vi "hotSpotsD2T.vi"(2 "Hotspot Number":i32, 3 "Basket Number":i32) -> (0 "rotation angle":dbl, 1 "distance to basket":dbl)   [LabVIEW 2011]
panel:
  # "z"
  # "R"
  # "Our Basket"
  # "yField"
  # "1"
  # "3"
  # "2"
  # "4"
  # "xField"
  # "xRobot"
  # "r"
  # "yRobot"
  # "y"
  # "x"
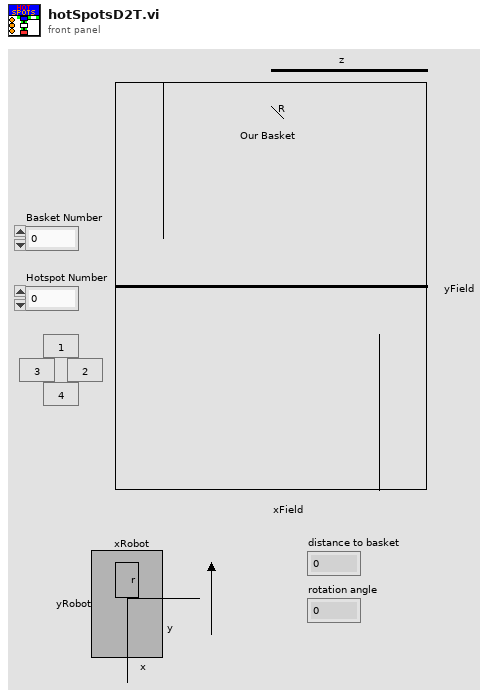
[diagram p1: front panel]
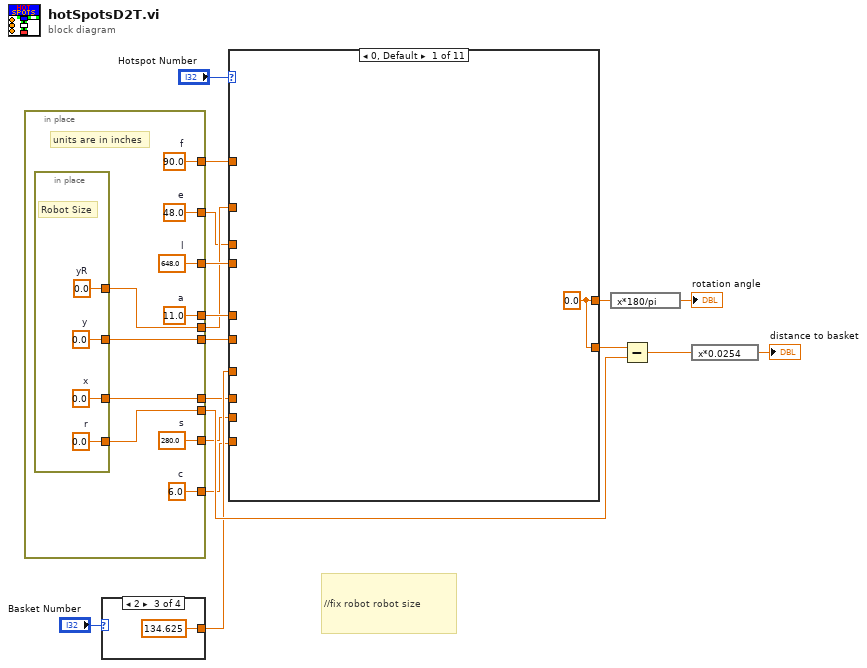
[diagram p0: block diagram]
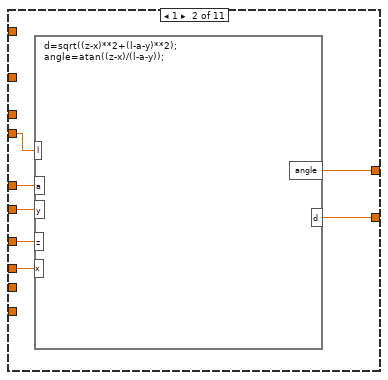
[diagram p2: hidden frame]
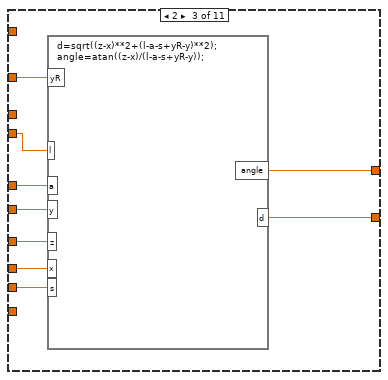
[diagram p3: hidden frame]
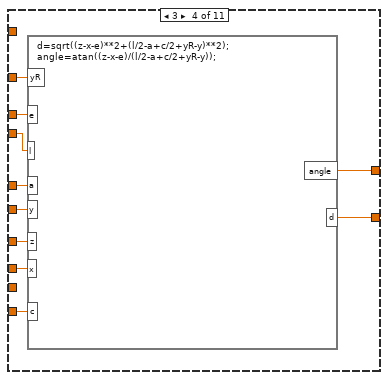
[diagram p4: hidden frame]
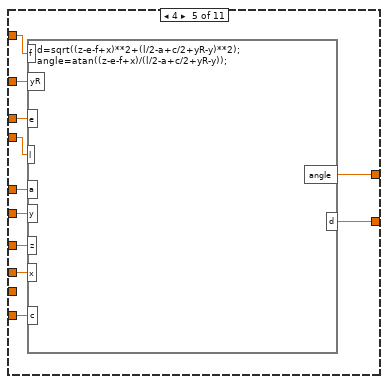
[diagram p5: hidden frame]
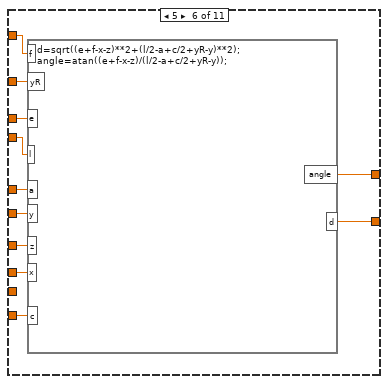
[diagram p6: hidden frame]
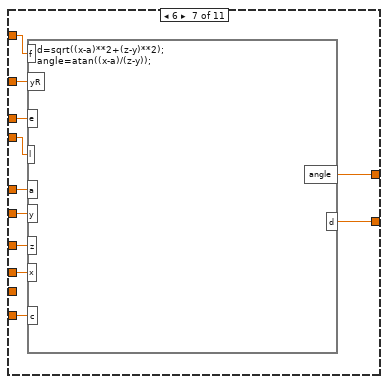
[diagram p7: hidden frame]
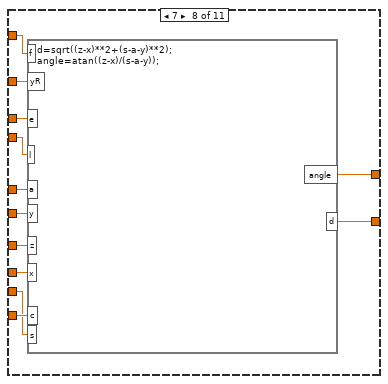
[diagram p8: hidden frame]
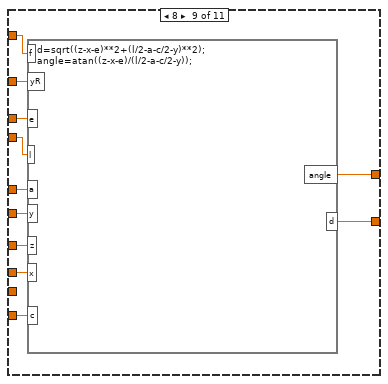
[diagram p9: hidden frame]
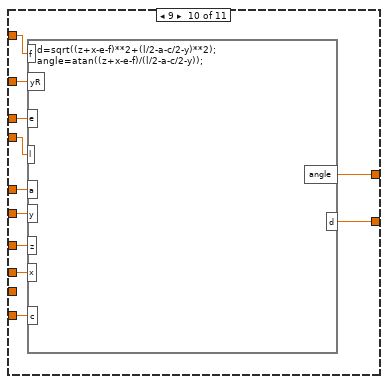
[diagram p10: hidden frame]
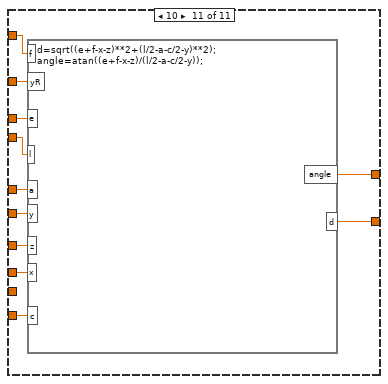
[diagram p11: hidden frame]
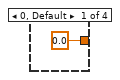
[diagram p12: hidden frame]
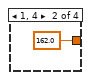
[diagram p13: hidden frame]
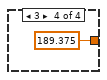
[diagram p14: hidden frame]
diagram:
  # "//fix robot robot size"
  n1 = in-place {
    in-place-border: [w28] -> w11
    in-place-border: [w27] -> w10
    in-place-border: [w26] -> w9
    in-place-border: [w25] -> w8
    in-place-border: [w24] -> w6
    in-place-border: [w23] -> w5
    in-place-border: [w22] -> w4
    in-place-border: [w21] -> w3
    in-place-border: [w20] -> w2
    in-place-border: [w19] -> w1
    w19 = 90.0  # f
    w21 = 6.0  # c
    w20 = 48.0  # e
    w23 = 280.0  # s
    w26 = 11.0  # a
    w27 = 648.0  # l
    # "units are in inches"
    n2 = in-place {
      in-place-border: [w32] -> w24
      in-place-border: [w31] -> w22
      in-place-border: [w30] -> w25
      in-place-border: [w29] -> w28
      w32 = 0.0  # x
      w30 = 0.0  # y
      w31 = 0.0  # yR
      w29 = 0.0  # r
      # "Robot Size"
    }
  }
  n3 = case shown="2" "Basket Number" {
    tunnel: [0.0 ("z") 162.0 ("z") 134.625 ("z") 189.375 ("z")] -> w7
    frame 0, Default {
    }
    frame 1, 4 {
    }
    frame 2 {
    }
    frame 3 {
    }
  }
  n4 = case shown="0, Default" "Hotspot Number" {
    tunnel: [w37 w44 w53 w63 w74 w85 w96 w108 w119 w130 w141] -> w13
    tunnel: [w37 w43 w52 w62 w73 w84 w95 w107 w118 w129 w140] -> w12
    tunnel: w10 -> [_ w42 w51 w61 w72 w83 w94 w106 w117 w128 w139]
    tunnel: w9 -> [_ w41 w50 w60 w71 w82 w93 w105 w116 w127 w138]
    tunnel: w8 -> [_ w40 w49 w59 w70 w81 w92 w104 w115 w126 w137]
    tunnel: w7 -> [_ w39 w48 w58 w69 w80 w91 w103 w114 w125 w136]
    tunnel: w6 -> [_ w38 w47 w57 w68 w79 w90 w102 w113 w124 w135]
    tunnel: w5 -> [_ _ w46 _ _ _ _ w97 _ _ _]
    tunnel: w4 -> [_ _ w45 w56 w67 w78 w89 w101 w112 w123 w134]
    tunnel: w3 -> [_ _ _ w55 w66 w77 w88 w100 w111 w122 w133]
    tunnel: w2 -> [_ _ _ w54 w65 w76 w87 w99 w110 w121 w132]
    tunnel: w1 -> [_ _ _ _ w64 w75 w86 w98 w109 w120 w131]
    frame 0, Default {
      w37 = 0.0 ("angle")
    }
    frame 1 {
      n5 = formula code="d=sqrt((z-x)**2+(l-a-y)**2);\nangle=atan((z-x)/(l-a-y));"("l"=w42, "z"=w39, "a"=w41, "x"=w38, "y"=w40) -> ("d"=w44:dbl, "angle"=w43:dbl)
    }
    frame 2 {
      n6 = formula code="d=sqrt((z-x)**2+(l-a-s+yR-y)**2);\nangle=atan((z-x)/(l-a-s+yR-y));"("l"=w51, "z"=w48, "a"=w50, "x"=w47, "y"=w49, "s"=w46, "yR"=w45) -> ("d"=w53:dbl, "angle"=w52:dbl)
    }
    frame 3 {
      n7 = formula code="d=sqrt((z-x-e)**2+(l/2-a+c/2+yR-y)**2);\nangle=atan((z-x-e)/(l/2-a+c/2+yR-y));"("l"=w61, "z"=w58, "a"=w60, "x"=w57, "y"=w59, "c"=w55, "yR"=w56, "e"=w54) -> ("d"=w63:dbl, "angle"=w62:dbl)
    }
    frame 4 {
      n8 = formula code="d=sqrt((z-e-f+x)**2+(l/2-a+c/2+yR-y)**2);\nangle=atan((z-e-f+x)/(l/2-a+c/2+yR-y));"("l"=w72, "z"=w69, "a"=w71, "x"=w68, "y"=w70, "c"=w66, "yR"=w67, "e"=w65, "f"=w64) -> ("d"=w74:dbl, "angle"=w73:dbl)
    }
    frame 5 {
      n9 = formula code="d=sqrt((e+f-x-z)**2+(l/2-a+c/2+yR-y)**2);\nangle=atan((e+f-x-z)/(l/2-a+c/2+yR-y));"("l"=w83, "z"=w80, "a"=w82, "x"=w79, "y"=w81, "c"=w77, "yR"=w78, "e"=w76, "f"=w75) -> ("d"=w85:dbl, "angle"=w84:dbl)
    }
    frame 6 {
      n10 = formula code="d=sqrt((x-a)**2+(z-y)**2);\nangle=atan((x-a)/(z-y));"("l"=w94, "z"=w91, "a"=w93, "x"=w90, "y"=w92, "c"=w88, "yR"=w89, "e"=w87, "f"=w86) -> ("d"=w96:dbl, "angle"=w95:dbl)
    }
    frame 7 {
      n11 = formula code="d=sqrt((z-x)**2+(s-a-y)**2);\nangle=atan((z-x)/(s-a-y));"("l"=w106, "z"=w103, "a"=w105, "x"=w102, "y"=w104, "c"=w100, "yR"=w101, "e"=w99, "f"=w98, "s"=w97) -> ("d"=w108:dbl, "angle"=w107:dbl)
    }
    frame 8 {
      n12 = formula code="d=sqrt((z-x-e)**2+(l/2-a-c/2-y)**2);\nangle=atan((z-x-e)/(l/2-a-c/2-y));"("l"=w117, "z"=w114, "a"=w116, "x"=w113, "y"=w115, "c"=w111, "yR"=w112, "e"=w110, "f"=w109) -> ("d"=w119:dbl, "angle"=w118:dbl)
    }
    frame 9 {
      n13 = formula code="d=sqrt((z+x-e-f)**2+(l/2-a-c/2-y)**2);\nangle=atan((z+x-e-f)/(l/2-a-c/2-y));"("l"=w128, "z"=w125, "a"=w127, "x"=w124, "y"=w126, "c"=w122, "yR"=w123, "e"=w121, "f"=w120) -> ("d"=w130:dbl, "angle"=w129:dbl)
    }
    frame 10 {
      n14 = formula code="d=sqrt((e+f-x-z)**2+(l/2-a-c/2-y)**2);\nangle=atan((e+f-x-z)/(l/2-a-c/2-y));"("l"=w139, "z"=w136, "a"=w138, "x"=w135, "y"=w137, "c"=w133, "yR"=w134, "e"=w132, "f"=w131) -> ("d"=w141:dbl, "angle"=w140:dbl)
    }
  }
  n15 = expression code="x*180/pi"(w12) -> (→"rotation angle":dbl)
  n16 = Subtract(x=w13, y=w11) -> (x-y=w15:dbl)
  n17 = expression code="x*0.0254"(w15) -> (→"distance to basket":dbl)
